vi "DHE_SetBinning.vi"(0 "refnum":i32=2048, 7 "xbin":u16, 9 "ybin":u16, 11 "error in (no error)":errorcluster) -> (4 "fd out":i32, 6 "return value":i32, 8 "X total size":u16, 10 "Y total size":u16, 14 "DET_READ_TIME":sgl=3.5 format="%.2f", 15 "error out":errorcluster)   [LabVIEW 2016]
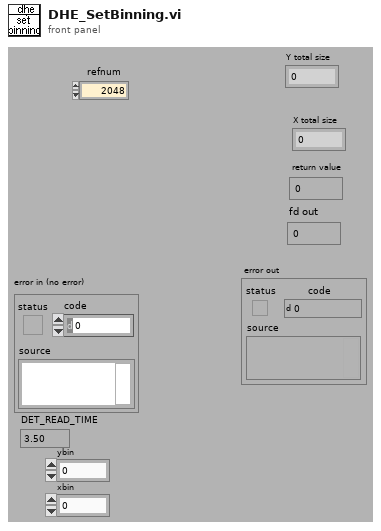
[diagram p1: front panel]
types:
  T1 = typedef "GEOM_CorrectedFPA.ctl" = cluster{"readmode":string, "amplifiers":cluster{"number":i32, "xstart":i32, "ystart":i32}[], "totxsize":i32, "totysize":i32, "maxxdim":i32, "maxydim":i32, "numxamps":i32, "numyamps":i32, "totxdata":i32, "totydata":i32, "xdataamp":i32, "ydataamp":i32, "totpixels":i32}
  T2 = typedef "GEOM_Amplifier.ctl" = cluster{"number":i32, "type":T3, "rotated":i16, "fliped":u16, "FPAcoord":cluster{"xstart":i32, "ystart":i32}, "Physical_size":cluster{"columns":i32, "rows":i32}, "predata":cluster{"columns":i32, "rows":i32}, "postdata":cluster{"columns":i32, "rows":i32}, "Req ROIs":T4, "Corr ROI":T4, "Detnumber":i32, "ampID":string, "discard":i32}
  T3 = typedef "GEOM_AmpType.ctl" = u16
  T4 = typedef "GEOM_ROI.ctl" = T5[]
  T5 = typedef "GEOM_Coords.ctl" = cluster{"xstart":u32, "ystart":u32, "xsize":u32, "ysize":u32}
  T6 = typedef "DatabaseHand_RefNum.ctl" = refnum<vi>
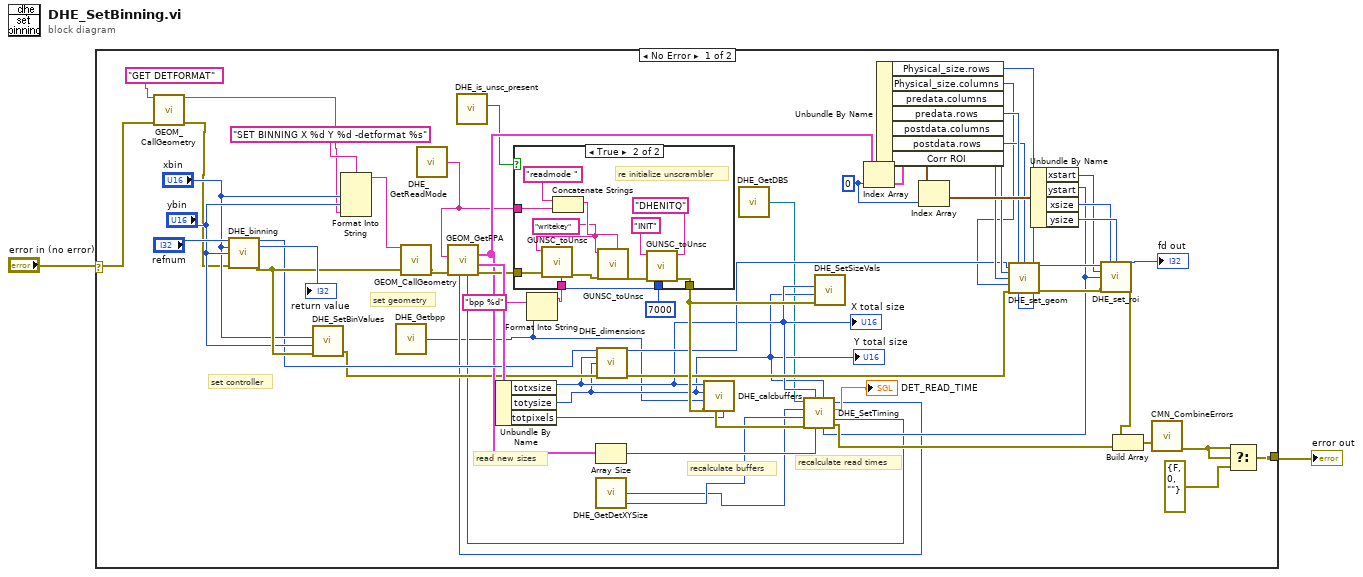
[diagram p0: block diagram]
diagram:
  n1 = case shown="No Error" "error in (no error)" {
    selector: "error in (no error)" -> [w5 w76]
    tunnel: [w43 w76] -> w2
    frame No Error {
      w41 = 0 ("index")
      # "recalculate read times"
      # "recalculate buffers"
      # "read new sizes"
      # "set geometry"
      # "set controller"
      n2 = call "GEOM_CallGeometry.vi"("Command"="GET DETFORMAT", "error in (no error)"=w5) -> ("ImmedReplyString"=w6:string, "error out"=w4:errorcluster)  [unwired: 12 out]
      n3 = call "DHE_binning.vi"("fd"="refnum", "xbin"="xbin", "ybin"="ybin", "error in (no error)"=w4) -> ("fd out"=w45:i32, "return value"=→"return value":i32, "error out"=w53:errorcluster)  [unwired: 9 out]
      n4 = call "DHE_SetBinValues.vi"("error in"=w53, "ybin"="ybin", "xbin"="xbin") -> ("errorout"=w25:errorcluster)  [unwired: 8 out]
      n5 = Format Into String(format string="SET BINNING X %d Y %d -detformat %s", "xbin", "ybin", w6) -> (resulting string=w60:string)  [unwired: 2 in, 1 out]
      n6 = call "DHE_Getbpp.vi"() -> ("DHE_bpp"=w11:i32)  [unwired: 9 out]
      n7 = call "GEOM_CallGeometry.vi"("Command"=w60, "error in (no error)"=w53) -> ("error out"=w56:errorcluster)  [unwired: 13 out]
      n8 = call "DHE_GetReadMode.vi"() -> ("DHE_ReadMode"=w12:string)  [unwired: 9 out]
      n9 = call "GEOM_GetFPA.vi"("error in (no error)"=w56, "readmode"=w12) -> ("error out"=w49:errorcluster, "CorrectedFPACoord"=w55:T1, "amplifiers"=w28:T2[], "numyamps"=w14:i32, "numxamps"=w15:i32)  [unwired: 1 in, 4 out]
      n10 = call "DHE_is_unsc_present.vi"() -> ("value"=w8:bool)  [unwired: 1 in, 10 out]
      n11 = Unbundle By Name(w55) -> ("totxsize"=w20:i32, "totysize"=w19:i32, "totpixels"=w7:i32)
      "Y total size" <- w19
      "X total size" <- w20
      n12 = Format Into String(format string="bpp %d", w11) -> (resulting string=w47:string)  [unwired: 2 in, 1 out]
      n13 = case shown="True" w8 {
        tunnel: [w63 w70] -> w50
        tunnel: w49 -> [w63 w69]
        tunnel: 7000 ("ms timeout (-1)") -> [_ w67]
        tunnel: w47 -> [_ w65]
        tunnel: w12 -> [_ w64]
        frame False {
        }
        frame True {
          w66 = "writekey" ("command")
          # "re initialize unscrambler"
          n14 = call "GUNSC_toUnsc.vi"("ms timeout (-1)"=w67, "key"=w65, "error in (no error)"=w69, "command"=w66) -> ("error out"=w68:errorcluster)  [unwired: 5 in, 2 out]
          n15 = Concatenate Strings("readmode " ("string"), w64) -> (w73:string)
          n16 = call "GUNSC_toUnsc.vi"("key"=w73, "error in (no error)"=w68, "command"=w66) -> ("error out"=w75:errorcluster)  [unwired: 6 in, 2 out]
          n17 = call "GUNSC_toUnsc.vi"("responseQ"="DHENITQ", "bpp"=w67, "error in (no error)"=w75, "command"="INIT") -> ("error out"=w70:errorcluster)  [unwired: 5 in, 2 out]
        }
      }
      n18 = Array Size(array=w28) -> (size(s)=w46:i32)
      n19 = call "DHE_GetDetXYSize.vi"() -> ("DHE_DetYsize"=w9:i32, "DHE_DetXsize"=w10:i32)  [unwired: 8 out]
      n20 = call "DHE_dimensions.vi"("fd"=w45, "Columns"=w20, "Rows"=w19, "error in (no error)"=w25) -> ("fd out"=w30:i32, "error out"=w27:errorcluster)  [unwired: 10 out]
      n21 = call "DHE_calcbuffers.vi"("totpixelsin"=w7, "error in (no error)"=w50, "bpp"=w11, "nrows"=w19, "ncols"=w20) -> ("error out"=w59:errorcluster)  [unwired: 1 in, 5 out]
      n22 = call "DHE_GetDBS.vi"() -> ("DHE_DBSRef"=w13:T6)  [unwired: 9 out]
      n23 = call "DHE_SetSizeVals.vi"("error in"=w50, "ytotsize"=w19, "xtotsize"=w20) -> ()  [unwired: 9 out]
      n24 = Index Array(array=w28, index=w41) -> (element=w40:T2)
      n25 = Unbundle By Name(w40) -> ("Physical_size.rows"=w17:i32, "Physical_size.columns"=w18:i32, "predata.columns"=w32:i32, "predata.rows"=w34:i32, "postdata.columns"=w31:i32, "postdata.rows"=w33:i32, "Corr ROI"=w39:T4)
      n26 = Index Array(array=w39, index=w41) -> (element=w38:T5)
      n27 = call "DHE_set_geom.vi"("fd"=w30, "ypredata"=w34, "ypostdata"=w33, "xpredata"=w32, "xpostdata"=w31, "xdata"=w18, "error in (no error)"=w27, "ydata"=w17) -> ("fd out"=w42:i32, "error out"=w26:errorcluster)  [unwired: 6 out]
      n28 = Unbundle By Name(w38) -> ("xstart"=w35:u32, "ystart"=w16:u32, "xsize"=w36:u32, "ysize"=w37:u32)
      n29 = call "DHE_SetTiming.vi"("num of Y amps"=w14, "num of X amps"=w15, "yroi start"=w16, "roi rows"=w19, "Num of amps"=w46, "roi cols"=w20, "error in"=w59, "totysize"=w10, "totxsize"=w9, "Database RefNum out"=w13) -> ("errorout"=w24:errorcluster, "DET_READ_TIME"=→"DET_READ_TIME":sgl)
      n30 = call "DHE_set_roi.vi"("fd"=w42, "xlenght"=w36, "ylenght"=w37, "xstart"=w35, "ystart"=w16, "error in (no error)"=w26) -> ("fd out"=→"fd out":i32, "error out"=w23:errorcluster)  [unwired: 8 out]
      n31 = Build Array(w23, w24) -> (w22:errorcluster[])
      n32 = call "CMN_CombineErrors.vi"("Errors"=w22) -> ("error out"=w21:errorcluster)  [unwired: 10 out]
      n33 = Select(t=w21, s=w21, f=errorcluster {"status"=FALSE, "code"=0, "source"=""}) -> (s? t:f=w43:errorcluster)
    }
    frame Error {
    }
  }
  "error out" <- w2
